vi "DeQ Valve Turbo State.vi"(8 "error in (no error)":errorcluster, 11 "Turbo in":refnum<class "Turbo.lvclass">) -> (0 "error out":errorcluster, 1 "timed out?":bool, 2 "State":u16, 3 "Turbo out":refnum<class "Turbo.lvclass">)   [LabVIEW 2015, in "cRIO-Carbondioxide.lvlib" / "CO2-Actor.lvlib" / "Turbo.lvclass"]
uses:
  Turbo.lvclass
  Turbo.lvclass/Turbo.ctl
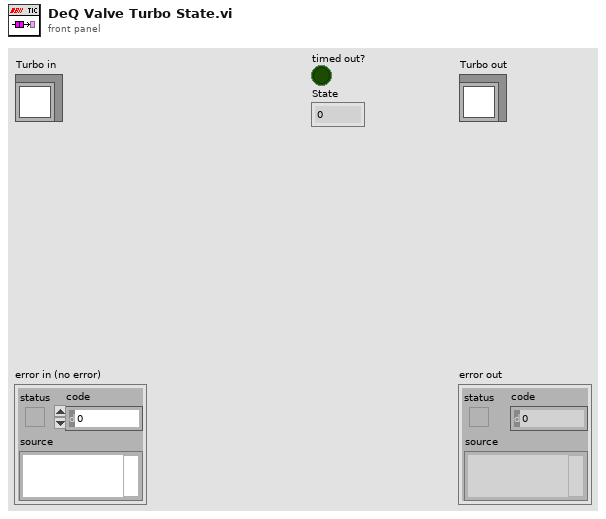
[diagram p1: front panel]
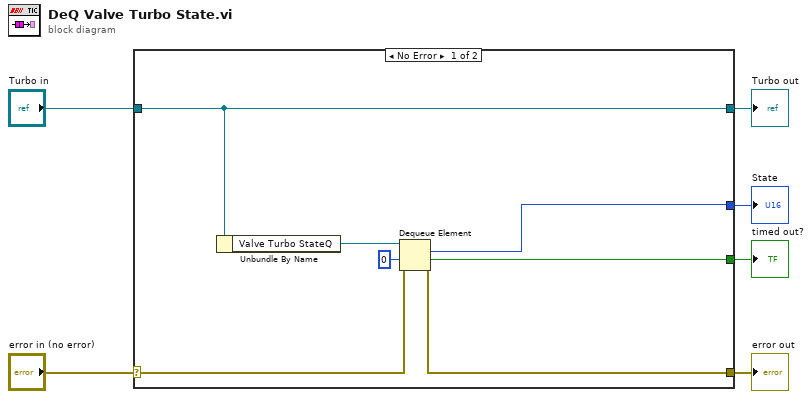
[diagram p0: block diagram]
diagram:
  n1 = case shown="No Error" "error in (no error)" {
    selector: "error in (no error)" -> [w11 w15]
    tunnel: [w10 w15] -> w5
    tunnel: [w13 w14] -> w3
    tunnel: "Turbo in" -> [w13 w14]
    tunnel: [w8 _] -> w1
    tunnel: [w7 _] -> w2
    frame No Error {
      n2 = Unbundle By Name(w13) -> ("Valve Turbo StateQ"=w12:refnum<queue>)
      n3 = Dequeue Element(queue=w12, timeout in ms (-1)=0, error in (no error)=w11) -> (element=w8:u16, timed out?=w7:bool, error out=w10:errorcluster)  [unwired: 1 out]
    }
    frame Error {
    }
  }
  "error out" <- w5
  "Turbo out" <- w3
  "timed out?" <- w2
  "State" <- w1
